vi "Ex8_ShiftRegister.vi"() -> ()   [LabVIEW 2024]
panel:
  out "number: 0 to 1":dbl
  in  "stop":bool
  out "0-1":dbl
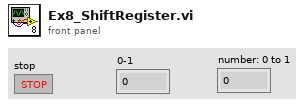
[diagram p1: front panel]
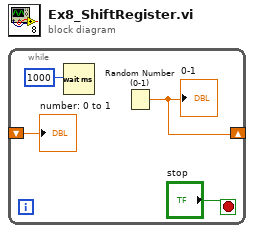
[diagram p0: block diagram]
diagram:
  n1 = while {
    shift-right: [w2] -> _
    shift-left: _ -> [w1]
    stop <- "stop" stop-if-true
    n2 = Wait (ms)(milliseconds to wait=1000) -> ()  [unwired: 1 out]
    n3 = Random Number (0-1)() -> (number: 0 to 1=w2:dbl)
    "0-1" <- w2
    "number: 0 to 1" <- w1
  }
